vi "Mock4.TestLauncher.vi"() -> ()   [LabVIEW 2016, in "Mock4.lvclass"]
uses:
  Mock4.lvclass
  <vilib>/JKI/JKI SMO/SMO/Typedefs/SMOState --Enum.ctl
  C:/Program Files (x86)/National Instruments/LabVIEW 2016/vi.lib/JKI/JKI SMO/SMO/SMO.lvclass
  C:/Program Files (x86)/National Instruments/LabVIEW 2016/vi.lib/JKI/JKI SMO/SMO.UI/SMO.UI.lvclass
  C:/Program Files (x86)/National Instruments/LabVIEW 2016/vi.lib/Levylab/Embedded SMO UI/EmbeddedSMO.lvclass
  <vilib>/JKI/JKI SMO/SMO/SMO.lvclass
  <vilib>/Levylab/Embedded SMO UI/EmbeddedSMO.lvclass
  <vilib>/JKI/JKI SMO/SMO.UI/SMO.UI.lvclass
panel:
  in  "Set Name?":bool
  in  "Write Name":string
  out "Read Name":string
  in  "Get Name?":bool
  out "SMO State":T1
  out "error out":errorcluster
  in  "Stop":bool
  # "Embedded SMO Test Launcher"
  # "For Debugging (Please Ignore)"
  # "For instructions on how to use the JKI State Machine Objects, examples and video tutorials, visit:\nhttp://jki.net/state-machine-objects/\n\nJKI State Machine Objects™\nhttp://jki.net/state-machine-objects/\nCopyright (C) 2005-2015, JKI <info@jki.net>\nALL RIGHTS RESERVED"
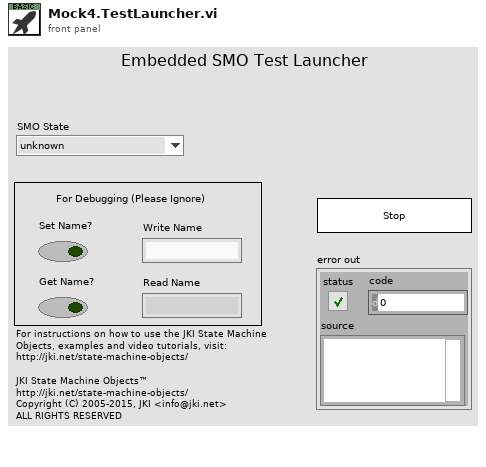
[diagram p1: front panel]
types:
  T1 = typedef "SMO.lvclass/SMOState --Enum.ctl" = enum16{"unknown", "Created", "Started", "Stopped"}
  T2 = typedef "SMO.lvclass/Public Events.ctl" = cluster{"Error":refnum<user-event>, "State":refnum<user-event>, "Reserve State":refnum<user-event>}
  T3 = cluster{"Event Registration Refnum":refnum<event-registration>}
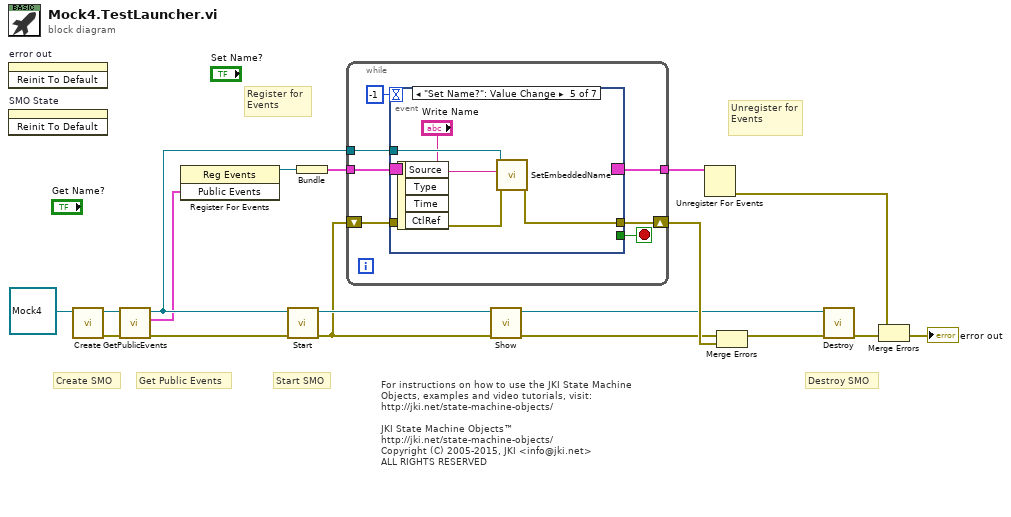
[diagram p0: block diagram]
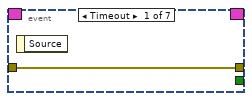
[diagram p2: hidden frame]
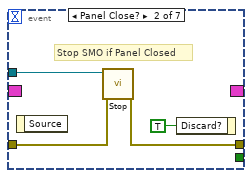
[diagram p3: hidden frame]
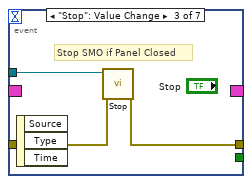
[diagram p4: hidden frame]
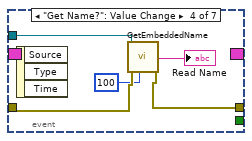
[diagram p5: hidden frame]
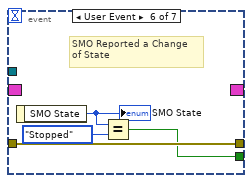
[diagram p6: hidden frame]
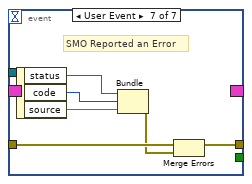
[diagram p7: hidden frame]
diagram:
  # "For instructions on how to use the JKI State Machine Objects, examples and video tutorials, visit:\nhttp://jki.net/state-machine-objects/\n\nJKI State Machine Objects™\nhttp://jki.net/state-machine-objects/\nCopyright (C) 2005-2015, JKI <info@jki.net>\nALL RIGHTS RESERVED"
  # "Get Public Events"
  # "Start SMO"
  # "Destroy SMO"
  # "Create SMO"
  # "Unregister for Events"
  # "Register for Events"
  n1 = invoke on="error out" class="Clust (strict)" method="Reinit To Default"() -> ()  [unwired: 3 in, 3 out]
  n2 = invoke on="SMO State" class="Enum (strict)" method="Reinit To Default"() -> ()  [unwired: 3 in, 3 out]
  n3 = call <vilib>:"Create.vi"("SMO"=refnum<class "Mock4.lvclass"> refnum ("SMO.Template.lvclass")) -> ("error out"=w9:errorcluster, "SMO out"=w10:refnum<class "Mock4.lvclass">)  [unwired: 8 in, 1 out]
  n4 = call <vilib>:"GetPublicEvents.vi"("error in (no error)"=w9, "SMO"=w10) -> ("error out"=w8:errorcluster, "Public Events"=w6:T2, "SMO out"=w7:refnum<class "Mock4.lvclass">)  [unwired: 7 in]
  n5 = register-events(w6) -> (reference out=w5:refnum<event-registration>)  [unwired: 2 in, 1 out]
  n6 = call <vilib>:"Start.vi"("error in (no error)"=w8, "SMO"=w7) -> ("error out"=w2:errorcluster, "SMO out"=w4:refnum<class "Mock4.lvclass">)  [unwired: 8 in]
  n7 = Bundle("Event Registration Refnum"=w5) -> (w17:T3)  [unwired: 1 in]
  n8 = while {
    shift-right: [w24] -> w16
    shift-left: w2 -> [w23]
    tunnel: w17 -> [w22]
    tunnel: [w21] -> w18
    tunnel: w7 -> [w20]
    stop <- w25 stop-if-true
    n9 = event shown="[4] \"Set Name?\": Value Change" {
      selector: w22 -> [_ _ _ _ _ _ _]
      dyn-events: [_ _ _ _ _ _ _] -> w21
      timeout: -1 -> [_ _ _ _ _ _ _]
      tunnel: [_ _ _ _ _ w43 _] -> w25
      tunnel: w20 -> [_ w30 w33 w38 w42 _ _]
      tunnel: [w26 w29 w32 w36 w39 w46 w50] -> w24
      tunnel: w23 -> [w26 w28 w31 w35 w40 w46 w48]
      event Timeout {
        n10 = event-data() -> ()  [unwired: 1 in, 1 out]
      }
      event Panel Close? {
        # "Stop SMO if Panel Closed"
        n11 = event-data() -> ()  [unwired: 1 in, 1 out]
        n12 = call <vilib>:"Stop.vi"("error in (no error)"=w28, "SMO"=w30) -> ("error out"=w29:errorcluster)  [unwired: 8 in, 1 out]
        n13 = event-data("Discard?"=TRUE ("OK")) -> ()  [unwired: 1 in, 1 out]
      }
      event "Stop": Value Change {
        # "Stop SMO if Panel Closed"
        n14 = event-data() -> ()  [unwired: 1 in, 3 out]
        n15 = call <vilib>:"Stop.vi"("error in (no error)"=w31, "SMO"=w33) -> ("error out"=w32:errorcluster)  [unwired: 8 in, 1 out]
      }
      event "Get Name?": Value Change {
        n16 = event-data() -> ()  [unwired: 1 in, 3 out]
        n17 = call <vilib>:"GetEmbeddedName.vi"("timeout in ms (-1)"=100, "error in (no error)"=w35, "EmbeddedSMO in"=w38) -> ("error out"=w36:errorcluster, "Name"=→"Read Name":string)  [unwired: 6 in, 1 out]
      }
      event "Set Name?": Value Change {
        n18 = event-data() -> ()  [unwired: 1 in, 4 out]
        n19 = call <vilib>:"SetEmbeddedName.vi"("error in (no error)"=w40, "Name"="Write Name", "EmbeddedSMO in"=w42) -> ("error out"=w39:errorcluster)  [unwired: 7 in, 1 out]
      }
      event User Event {
        # "SMO Reported a Change\nof State"
        n20 = event-data() -> ("SMO State"=w45:T1)  [unwired: 1 in]
        "SMO State" <- w45
        n21 = Equal?(x=w45, y=SMOState_--Enum."Stopped") -> (x = y?=w43:bool)
      }
      event User Event {
        # "SMO Reported an Error"
        n22 = event-data() -> ("status"=w49:bool, "code"=w52:i32, "source"=w51:string)  [unwired: 1 in]
        n23 = Bundle("status"=w49, "code"=w52, "source"=w51) -> (w47:errorcluster)  [unwired: 1 in]
        n24 = Merge Errors(w48, w47) -> (w50:errorcluster)
      }
    }
  }
  n25 = call <vilib>:"Show.vi"("error in (no error)"=w2, "SMO.UI"=w4) -> ("error out"=w1:errorcluster, "SMO.UI out"=w3:refnum<class "Mock4.lvclass">)  [unwired: 8 in]
  n26 = Unregister For Events(event registration refnum=w18) -> (error out=w15:errorcluster)  [unwired: 1 in]
  n27 = Merge Errors(w1, w16) -> (w11:errorcluster)
  n28 = call <vilib>:"Destroy.vi"("error in (no error)"=w11, "SMO"=w3) -> ("error out"=w13:errorcluster)  [unwired: 9 in]
  n29 = Merge Errors(w15, w13) -> (→"error out":errorcluster)
